vi "Climb.vi"() -> ()   [LabVIEW 2020]
uses:
  Team Code/Robot Global Data.vi
panel:
  in  "climberArmTolerance":dbl=250.0
  in  "climberWinchTolerance":dbl=5000.0
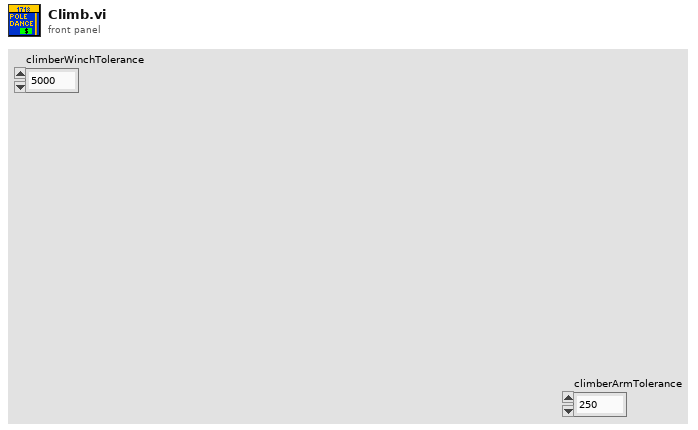
[diagram p1: front panel]
types:
  T1 = typedef "PiConfig.ctl" = cluster{"swerveModules":cluster{"leftFront":T2, "rightFront":T2, "leftRear":T2, "rightRear":T2}, "offsets":cluster{"leftFrontAngleOffset":dbl, "leftRearAngleOffset":dbl, "rightFrontAngleOffset":dbl, "rightRearAngleOffset":dbl}, "limits":cluster{"maxVelocity":dbl, "maxOverdriveVelocity":dbl, "maxAcceleration":dbl, "maxPickupVelocity":dbl}, "speeds":cluster{"intakeSuckSpeed":dbl, "intakeSpitSpeed":dbl, "indexerSuckSpeed":dbl, "indexerSpitSpeed":dbl, "indexerShootSpeed":dbl, "indexerBumpBackSpeed":dbl, "shooterSpinupSpeed":dbl, "kickupSpinupSpeed":dbl, "shooterLowShootSpeed":dbl, "shooterHighShootSpeed":dbl}, "positions":cluster{"intakeStarting":dbl, "intakeStow":dbl, "intakeSuck":dbl, "armPounce":dbl, "armStow":dbl, "armUp":dbl, "winchPounce":dbl, "winchOut":dbl, "winchStow":dbl, "intakeSpit":dbl, "winchBarEngage":dbl, "winchBottomClimb":dbl, "hoodHighShoot":dbl, "armAirOut":dbl, "armAirUp":dbl, "winchAirOut":dbl, "winchAirUp":dbl, "winchHighClimb":dbl, "winchTraversalClimb":dbl}, "inversions":cluster{"rightShooter":bool, "leftShooter":bool}}
  T2 = typedef "Swerve Module Parameters.ctl" = cluster{"driveCANID":dbl, "angleCANID":i32, "canCoderCANID":dbl, "moduleName":string, "driveMotorNeutralMode":T3, "driveCurrentLimitConfig":T4, "driveFeedbackDevice":T5, "driveInitialSensorPosition":dbl, "driveEnableVoltageComp":bool, "driveVoltageComp":dbl, "driveRampRate":dbl, "angleCurrentLimit":dbl, "angleSensorType":T6, "angleMotorType":T7, "angleConversionFactor":dbl, "anglePIDRamp":dbl, "angleVoltageComp":dbl, "angleIdleMode":T8, "cancoderConfig":T9, "angleInitialSensorPosition":dbl}
  T3 = typedef "CTRE_Phoenix_MotorControl_NeutralMode.ctl" = enum8{"EEPROMSetting", "Override to Coast", "Override to Brake"}
  T4 = typedef "CTRE_Phoenix_MotorControl_SupplyCurrentLimitConfiguration.ctl" = cluster{"Enable?":bool, "Current Limit":dbl, "Threshold Current":dbl, "Threshold Time":dbl}
  T5 = typedef "CTRE_Phoenix_MotorControl_FeedbackDevice_TalonFX.ctl" = i8
  T6 = typedef "Spark MAX Sensor Type.ctl" = enum16{"No Sensor", "Hall Sensor", "Encoder", "-Not Available-", "Analog", "Alternate Encoder"}
  T7 = typedef "Spark MAX Motor Type.ctl" = enum16{"Brushed", "Brushless"}
  T8 = typedef "Spark MAX Idle Mode.ctl" = enum16{"Coast", "Brake"}
  T9 = typedef "CTRE_Phoenix_CANcoder_Configurables.ctl" = cluster{"Sensor Initialization Strategy":T10, "Absolute Sensor Range":T11, "Velocity Measurement Period":T12, "Velocity Measurement Window":i32, "Magnet Offset (Degrees)":dbl, "Sensor Direction":bool, "Sensor Coefficient":dbl, "Unit String":string, "Sensor Time Base":T13}
  T10 = typedef "CTRE_Phoenix_CANcoder_SensorInitializationStrategy.ctl" = enum16{"Boot To Zero", "Boot To Absolute Position"}
  T11 = typedef "CTRE_Phoenix_CANcoder_AbsoluteSensorRange.ctl" = enum16{"Unsigned [0 to 360)", "Signed [-180 to +180)"}
  T12 = typedef "CTRE_Phoenix_MotorControl_VelocityMeasurementPeriod.ctl" = u16
  T13 = typedef "CTRE_Phoenix_CANcoder_SensorTimeBase.ctl" = enum16{"Per100Ms_Legacy", "PerSecond", "PerMinute"}
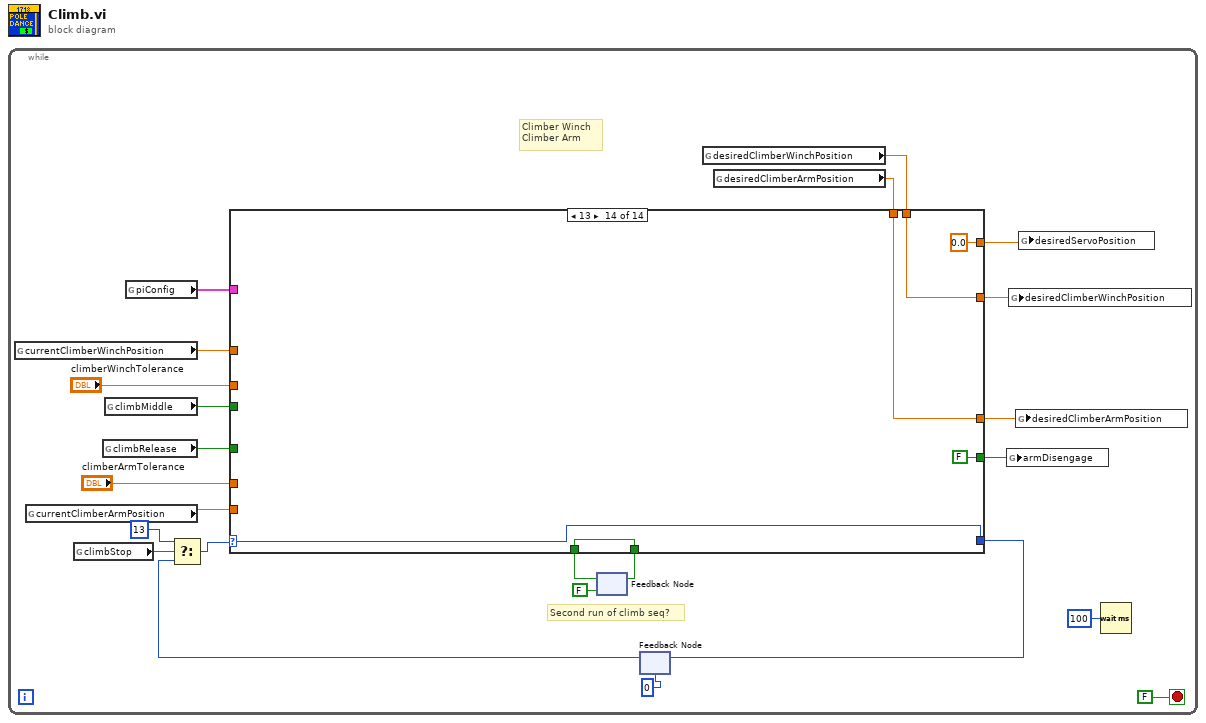
[diagram p0: block diagram]
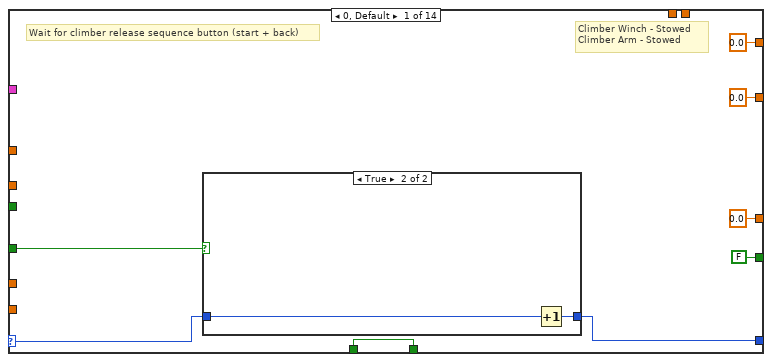
[diagram p2: hidden frame]
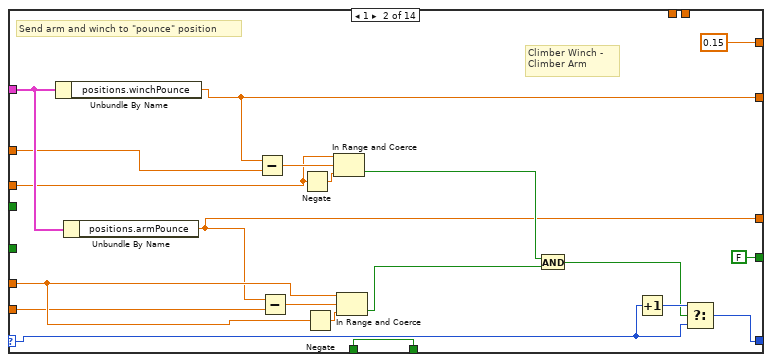
[diagram p4: hidden frame]
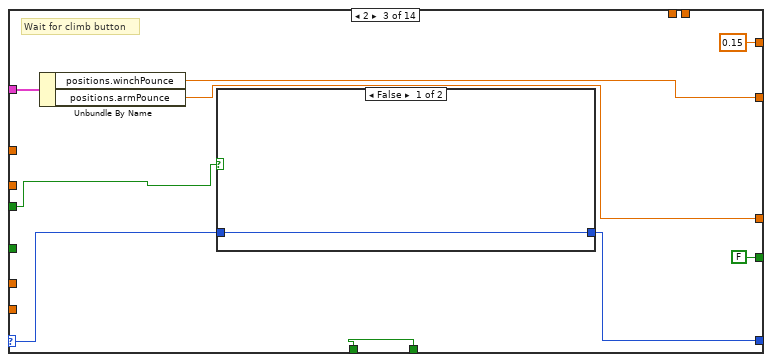
[diagram p5: hidden frame]
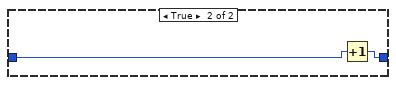
[diagram p6: hidden frame]
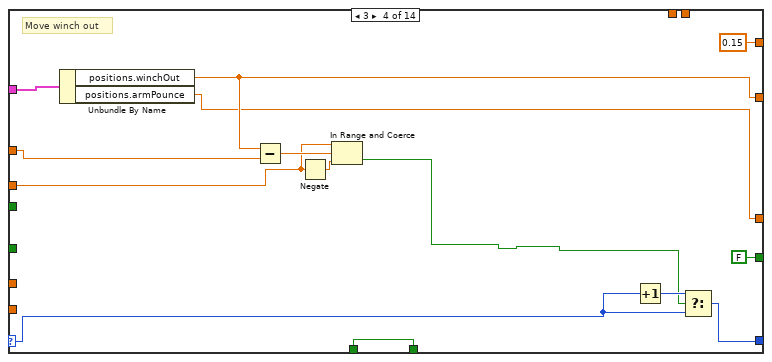
[diagram p7: hidden frame]
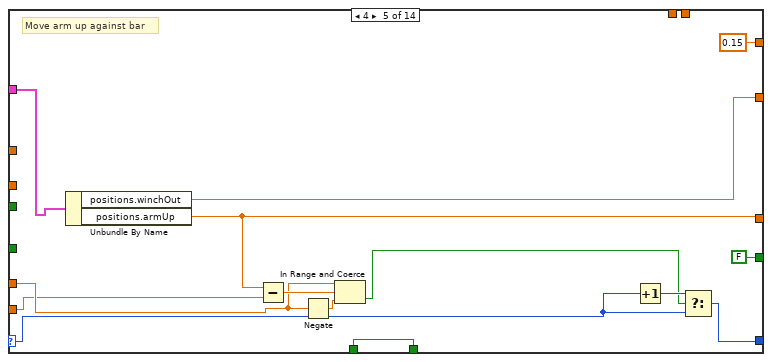
[diagram p8: hidden frame]
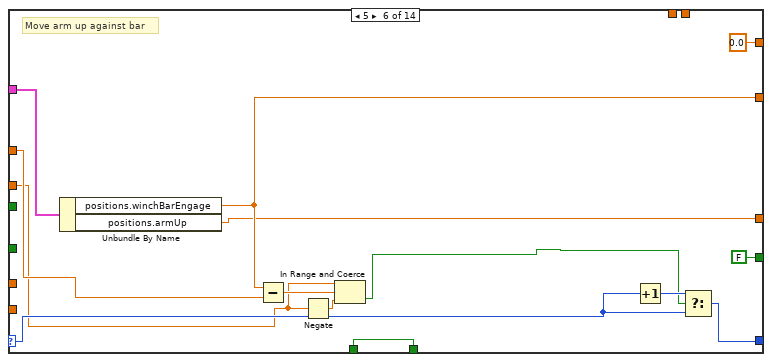
[diagram p9: hidden frame]
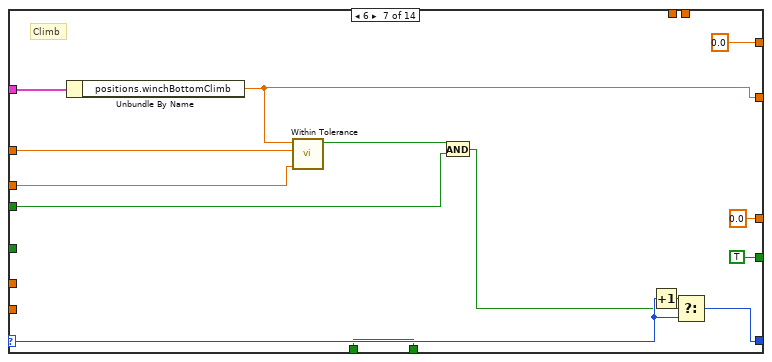
[diagram p10: hidden frame]
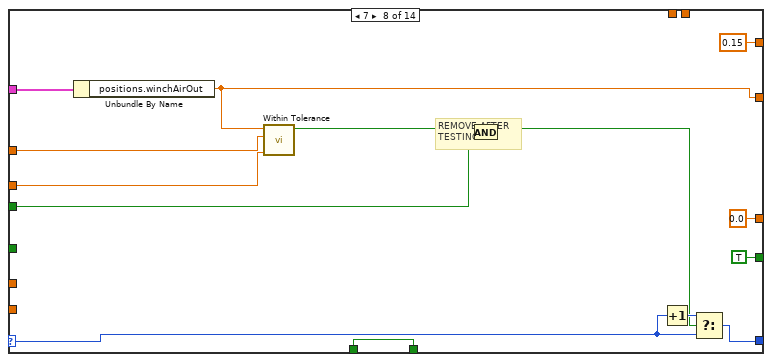
[diagram p11: hidden frame]
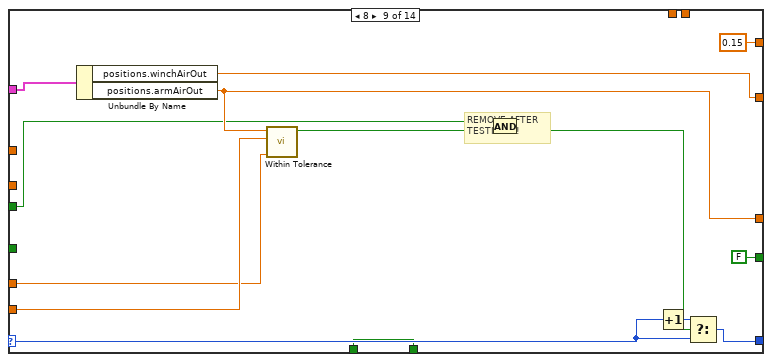
[diagram p12: hidden frame]
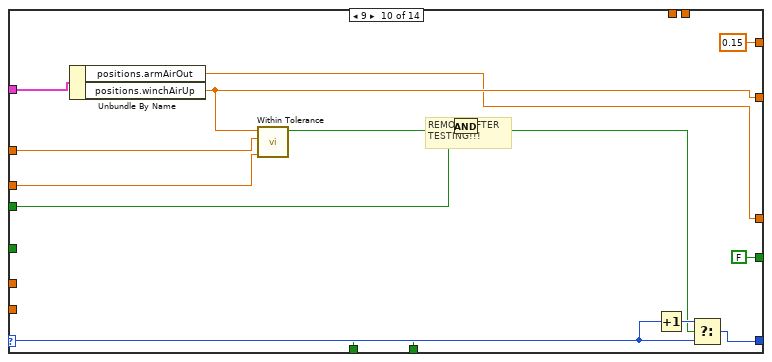
[diagram p13: hidden frame]
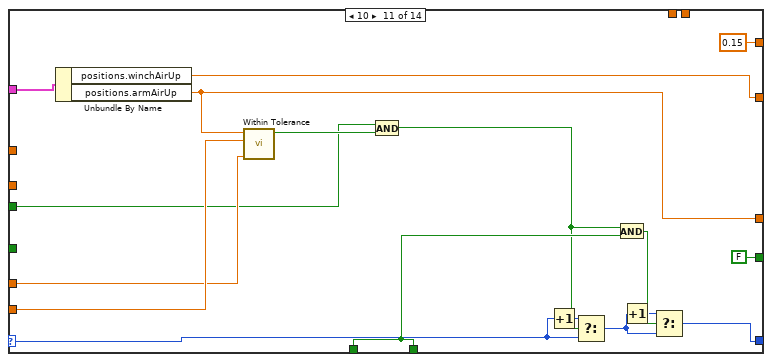
[diagram p14: hidden frame]
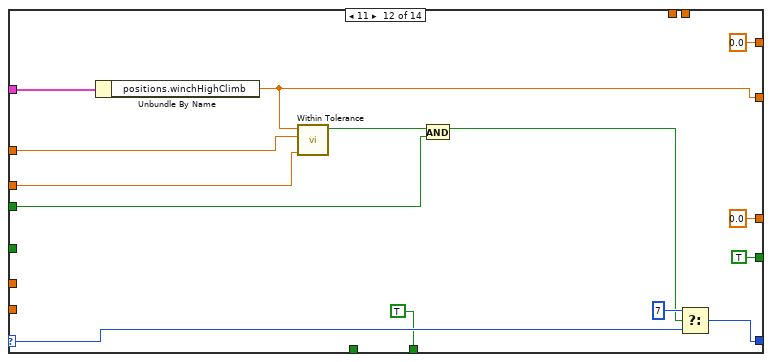
[diagram p15: hidden frame]
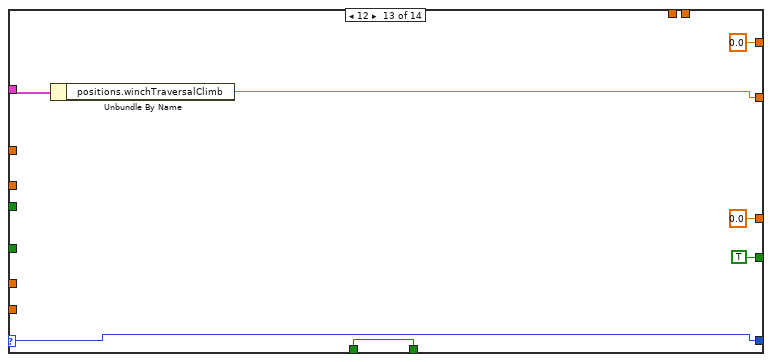
[diagram p16: hidden frame]
diagram:
  n1 = while {
    stop <- FALSE stop-if-true
    # "Second run of climb seq?"
    # "Climber Winch\nClimber Arm"
    n2 = global read "Robot Global Data.vi" "currentClimberWinchPosition"() -> (w17:dbl)
    n3 = global read "Robot Global Data.vi" "currentClimberArmPosition"() -> (w13:dbl)
    n4 = global read "Robot Global Data.vi" "climbStop"() -> (w3:bool)
    n5 = global read "Robot Global Data.vi" "climbRelease"() -> (w18:bool)
    n6 = global read "Robot Global Data.vi" "climbMiddle"() -> (w10:bool)
    n7 = global read "Robot Global Data.vi" "piConfig"() -> (w22:T1)
    n8 = feedback #1(FALSE) -> (w8:bool)
    n9 = feedback #2(0) -> (w4:i32)
    n10 = Select(t=13, s=w3, f=w4) -> (s? t:f=w2:i32)
    n11 = global read "Robot Global Data.vi" "desiredClimberWinchPosition"() -> (w6:dbl)
    n12 = global read "Robot Global Data.vi" "desiredClimberArmPosition"() -> (w5:dbl)
    n13 = case shown="13" w2 {
      selector: w2 -> [w31 w43 w63 w75 w89 w104 w116 w130 w148 w160 w178 w194 w197 w205]
      tunnel: [w32 w52 w64 w76 w90 w105 w117 w131 w149 w161 w171 w195 w197 w205] -> w23
      tunnel: w22 -> [_ w49 w61 w78 w92 w106 w123 w136 w151 w165 w182 w196 w203 _]
      tunnel: "climberWinchTolerance" -> [_ w45 _ w77 _ w97 w112 w127 _ w163 _ w192 _ _]
      tunnel: "climberArmTolerance" -> [_ w44 _ _ w91 _ _ _ w145 _ w180 _ _ _]
      tunnel: w18 -> [w30 _ _ _ _ _ _ _ _ _ _ _ _ _]
      tunnel: w17 -> [_ w42 _ w74 _ w98 w118 w135 _ w164 _ w193 _ _]
      tunnel: [0.0 ("winchOut") w41 w60 w73 w85 w101 w119 w134 w140 w162 w169 w190 w200 w209] -> w16
      tunnel: [0.0 ("desiredServoPosition") 0.15 ("desiredServoPosition") 0.15 ("desiredServoPosition") 0.15 ("desiredServoPosition") 0.15 ("desiredServoPosition") 0.0 ("desiredServoPosition") 0.0 ("desiredServoPosition") 0.15 ("desiredServoPosition") 0.15 ("desiredServoPosition") 0.15 ("desiredServoPosition") 0.15 ("desiredServoPosition") 0.0 ("desiredServoPosition") 0.0 ("desiredServoPosition") 0.0 ("desiredServoPosition")] -> w15
      tunnel: [0.0 ("armUp") w39 w59 w71 w88 w100 0.0 ("armUp") 0.0 ("armUp") w143 w155 w179 0.0 ("armAirUp") 0.0 ("armAirUp") w208] -> w14
      tunnel: w13 -> [_ w38 _ _ w86 _ _ _ w150 _ w181 _ _ _]
      tunnel: w10 -> [_ _ w56 _ _ _ w110 w124 w138 w152 w166 w183 _ _]
      tunnel: [FALSE ("armDisengage") FALSE ("armDisengage") FALSE ("armDisengage") FALSE ("armDisengage") FALSE ("armDisengage") FALSE ("armDisengage") TRUE ("armDisengage") TRUE ("armDisengage") FALSE ("armDisengage") FALSE ("armDisengage") FALSE ("armDisengage") TRUE ("armDisengage") TRUE ("armDisengage") FALSE ("armDisengage")] -> w12
      tunnel: [w25 w36 w57 w68 w82 w96 w111 w126 w142 w156 w175 TRUE w202 w204] -> w9
      tunnel: w8 -> [w25 w36 w57 w68 w82 w96 w111 w126 w142 w156 w175 _ w202 w204]
      tunnel: w6 -> [_ _ _ _ _ _ _ _ _ _ _ _ _ w209]
      tunnel: w5 -> [_ _ _ _ _ _ _ _ _ _ _ _ _ w208]
      frame 0, Default {
        # "Climber Winch - Stowed\nClimber Arm - Stowed"
        # "Wait for climber release sequence button (start + back)"
        n14 = case shown="True" w30 {
          tunnel: w31 -> [w33 w34]
          tunnel: [w33 w35] -> w32
          frame False {
          }
          frame True {
            n15 = Increment(x=w34) -> (x+1=w35:i32)
          }
        }
      }
      frame 1 {
        # "Climber Winch - \nClimber Arm"
        # "Send arm and winch to \"pounce\" position"
        n16 = Unbundle By Name(w49) -> ("positions.winchPounce"=w41:dbl)
        n17 = Unbundle By Name(w49) -> ("positions.armPounce"=w39:dbl)
        n18 = Subtract(x=w41, y=w42) -> (x-y=w55:dbl)
        n19 = Subtract(x=w39, y=w38) -> (x-y=w51:dbl)
        n20 = Negate(x=w45) -> (-x=w54:dbl)
        n21 = Negate(x=w44) -> (-x=w50:dbl)
        n22 = In Range and Coerce(upper limit=w45, x=w55, lower limit=w54) -> (In Range?=w48:bool)  [unwired: 1 out]
        n23 = In Range and Coerce(upper limit=w44, x=w51, lower limit=w50) -> (In Range?=w47:bool)  [unwired: 1 out]
        n24 = And(x=w48, y=w47) -> (x .and. y?=w46:bool)
        n25 = Increment(x=w43) -> (x+1=w53:i32)
        n26 = Select(t=w53, s=w46, f=w43) -> (s? t:f=w52:i32)
      }
      frame 2 {
        # "Wait for climb button"
        n27 = Unbundle By Name(w61) -> ("positions.winchPounce"=w60:dbl, "positions.armPounce"=w59:dbl)
        n28 = case shown="False" w56 {
          tunnel: w63 -> [w65 w66]
          tunnel: [w65 w67] -> w64
          frame False {
          }
          frame True {
            n29 = Increment(x=w66) -> (x+1=w67:i32)
          }
        }
      }
      frame 3 {
        # "Move winch out"
        n30 = Unbundle By Name(w78) -> ("positions.winchOut"=w73:dbl, "positions.armPounce"=w71:dbl)
        n31 = Subtract(x=w73, y=w74) -> (x-y=w81:dbl)
        n32 = Negate(x=w77) -> (-x=w80:dbl)
        n33 = In Range and Coerce(upper limit=w77, x=w81, lower limit=w80) -> (In Range?=w69:bool)  [unwired: 1 out]
        n34 = Increment(x=w75) -> (x+1=w79:i32)
        n35 = Select(t=w79, s=w69, f=w75) -> (s? t:f=w76:i32)
      }
      frame 4 {
        # "Move arm up against bar"
        n36 = Unbundle By Name(w92) -> ("positions.winchOut"=w85:dbl, "positions.armUp"=w88:dbl)
        n37 = Subtract(x=w88, y=w86) -> (x-y=w94:dbl)
        n38 = Negate(x=w91) -> (-x=w93:dbl)
        n39 = In Range and Coerce(upper limit=w91, x=w94, lower limit=w93) -> (In Range?=w83:bool)  [unwired: 1 out]
        n40 = Increment(x=w89) -> (x+1=w95:i32)
        n41 = Select(t=w95, s=w83, f=w89) -> (s? t:f=w90:i32)
      }
      frame 5 {
        # "Move arm up against bar"
        n42 = Unbundle By Name(w106) -> ("positions.winchBarEngage"=w101:dbl, "positions.armUp"=w100:dbl)
        n43 = Subtract(x=w101, y=w98) -> (x-y=w108:dbl)
        n44 = Negate(x=w97) -> (-x=w107:dbl)
        n45 = In Range and Coerce(upper limit=w97, x=w108, lower limit=w107) -> (In Range?=w102:bool)  [unwired: 1 out]
        n46 = Increment(x=w104) -> (x+1=w109:i32)
        n47 = Select(t=w109, s=w102, f=w104) -> (s? t:f=w105:i32)
      }
      frame 6 {
        # "Climb"
        n48 = Unbundle By Name(w123) -> ("positions.winchBottomClimb"=w119:dbl)
        n49 = call "Within Tolerance.vi"("tolerance"=w112, "input"=w118, "target"=w119) -> ("withinTolerance"=w114:bool)  [unwired: 8 in]
        n50 = And(x=w114, y=w110) -> (x .and. y?=w113:bool)
        n51 = Increment(x=w116) -> (x+1=w115:i32)
        n52 = Select(t=w115, s=w113, f=w116) -> (s? t:f=w117:i32)
      }
      frame 7 {
        # "REMOVE AFTER\nTESTING!!!"
        n53 = Unbundle By Name(w136) -> ("positions.winchAirOut"=w134:dbl)
        n54 = call "Within Tolerance.vi"("tolerance"=w127, "input"=w135, "target"=w134) -> ("withinTolerance"=w129:bool)  [unwired: 8 in]
        n55 = And(x=w129, y=w124) -> (x .and. y?=w125:bool)
        n56 = Increment(x=w130) -> (x+1=w128:i32)
        n57 = Select(t=w128, s=w125, f=w130) -> (s? t:f=w131:i32)
      }
      frame 8 {
        # "REMOVE AFTER\nTESTING!!!"
        n58 = Unbundle By Name(w151) -> ("positions.winchAirOut"=w140:dbl, "positions.armAirOut"=w143:dbl)
        n59 = call "Within Tolerance.vi"("tolerance"=w145, "input"=w150, "target"=w143) -> ("withinTolerance"=w146:bool)  [unwired: 8 in]
        n60 = And(x=w138, y=w146) -> (x .and. y?=w139:bool)
        n61 = Increment(x=w148) -> (x+1=w147:i32)
        n62 = Select(t=w147, s=w139, f=w148) -> (s? t:f=w149:i32)
      }
      frame 9 {
        # "REMOVE AFTER\nTESTING!!!"
        n63 = Unbundle By Name(w165) -> ("positions.armAirOut"=w155:dbl, "positions.winchAirUp"=w162:dbl)
        n64 = call "Within Tolerance.vi"("tolerance"=w163, "input"=w164, "target"=w162) -> ("withinTolerance"=w158:bool)  [unwired: 8 in]
        n65 = And(x=w152, y=w158) -> (x .and. y?=w153:bool)
        n66 = Increment(x=w160) -> (x+1=w159:i32)
        n67 = Select(t=w159, s=w153, f=w160) -> (s? t:f=w161:i32)
      }
      frame 10 {
        n68 = Unbundle By Name(w182) -> ("positions.winchAirUp"=w169:dbl, "positions.armAirUp"=w179:dbl)
        n69 = call "Within Tolerance.vi"("tolerance"=w180, "input"=w181, "target"=w179) -> ("withinTolerance"=w176:bool)  [unwired: 8 in]
        n70 = And(x=w166, y=w176) -> (x .and. y?=w167:bool)
        n71 = Increment(x=w178) -> (x+1=w177:i32)
        n72 = Select(t=w177, s=w167, f=w178) -> (s? t:f=w173:i32)
        n73 = And(x=w167, y=w175) -> (x .and. y?=w174:bool)
        n74 = Increment(x=w173) -> (x+1=w172:i32)
        n75 = Select(t=w172, s=w174, f=w173) -> (s? t:f=w171:i32)
      }
      frame 11 {
        n76 = Unbundle By Name(w196) -> ("positions.winchHighClimb"=w190:dbl)
        n77 = call "Within Tolerance.vi"("tolerance"=w192, "input"=w193, "target"=w190) -> ("withinTolerance"=w187:bool)  [unwired: 8 in]
        n78 = And(x=w187, y=w183) -> (x .and. y?=w184:bool)
        n79 = Select(t=7, s=w184, f=w194) -> (s? t:f=w195:i32)
      }
      frame 12 {
        n80 = Unbundle By Name(w203) -> ("positions.winchTraversalClimb"=w200:dbl)
      }
      frame 13 {
      }
    }
    n81 = feedback-in #1(w9) -> ()
    n82 = feedback-in #2(w23) -> ()
    n83 = global write "Robot Global Data.vi" "armDisengage"(w12) -> ()
    n84 = global write "Robot Global Data.vi" "desiredClimberWinchPosition"(w16) -> ()
    n85 = global write "Robot Global Data.vi" "desiredClimberArmPosition"(w14) -> ()
    n86 = global write "Robot Global Data.vi" "desiredServoPosition"(w15) -> ()
    n87 = Wait (ms)(milliseconds to wait=u32 100) -> ()  [unwired: 1 out]
  }
